vi "Sort Gannt Chart.vi"(10 "Gannt Chart  in":T1[][](array[typedef]), 11 "Machine Number":i32) -> (3 "Gannt Chart Out out":T1[][](array[typedef]))   [LabVIEW 2013, in "GA.lvclass"]
uses:
  GA.lvclass
  Controls/GanntChart_Element.ctl
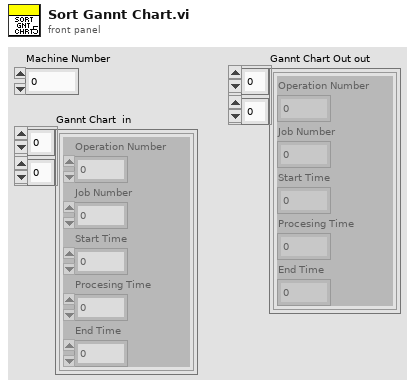
[diagram p1: front panel]
types:
  T1 = typedef "GanntChart_Element.ctl" = cluster{"Operation Number":i32, "Job Number":i32, "Start Time":i32, "Procesing Time":u16, "End Time":i32}
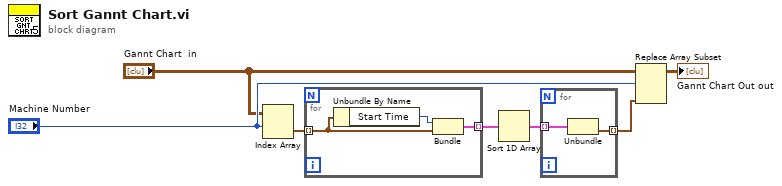
[diagram p0: block diagram]
diagram:
  n1 = Index Array(array="Gannt Chart  in", index (row)="Machine Number") -> (element=w4:T1[])  [unwired: 1 in]
  n2 = for {
    tunnel: w4 -> [w9] mode=indexing
    tunnel: [w8] -> w3 mode=indexing
    n3 = Unbundle By Name(w9) -> ("Start Time"=w10:i32)
    n4 = Bundle("Start Time"=w10, w9) -> (w8:cluster{"Start Time":i32, T1})  [unwired: 1 in]
  }
  n5 = Sort 1D Array(array=w3) -> (sorted array=w2:cluster{"Start Time":i32, T1}[])
  n6 = for {
    tunnel: w2 -> [w12] mode=indexing
    tunnel: [w11] -> w1 mode=indexing
    n7 = Unbundle(w12) -> (w11:T1)  [unwired: 1 out]
  }
  n8 = Replace Array Subset(array="Gannt Chart  in", new element=w1, index (row)="Machine Number") -> (→"Gannt Chart Out out":T1[][])  [unwired: 1 in]
